vi "Morse Code Decoder.vi"(8 "error in":errorcluster, 10 "Map":map{string, string}(c390), 11 "Message to Decode":string) -> (0 "error out":errorcluster, 3 "Decoded Array":string[](array[string]))   [LabVIEW 2022 SP3]
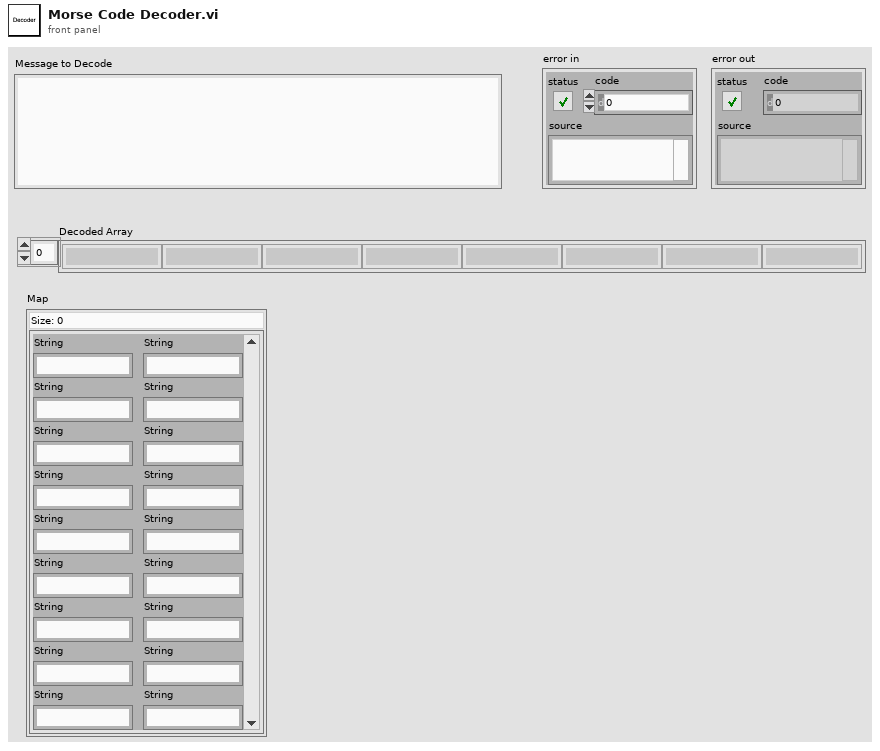
[diagram p1: front panel]
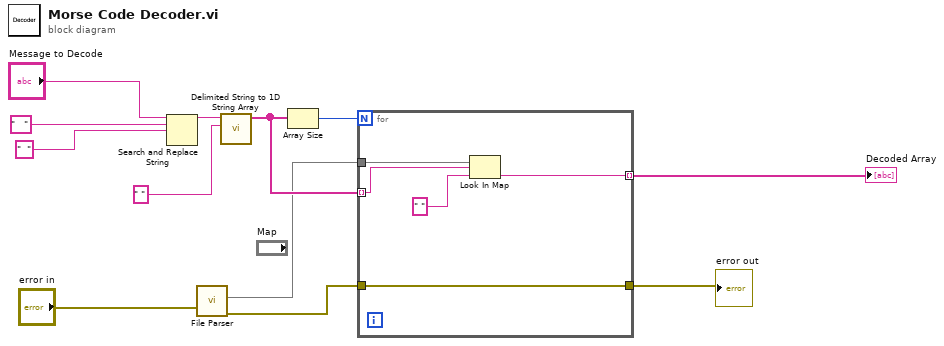
[diagram p0: block diagram]
diagram:
  n1 = Search and Replace String(input string="Message to Decode", search string="   " ("substring (\"\")"), replace string="  " ("replace string (\"\")")) -> (result string=w8:string)  [unwired: 5 in, 3 out]
  n2 = call "File Parser.vi"("error in (no error)"="error in") -> ("error out"=w3:errorcluster, "Morse-Letter Map (output 2)"=w4:map{string, string})  [unwired: 8 in, 1 out]
  n3 = call <vilib>:"Delimited String to 1D String Array.vi"("delimiter"=" ", "delimited string"=w8) -> ("string array"=w6:string[])  [unwired: 9 in]
  n4 = Array Size(array=w6) -> (size(s)=w7:i32)
  n5 = for {
    N: w7 -> [_]
    tunnel: w4 -> [w17]
    tunnel: w6 -> [w16] mode=indexing
    tunnel: [w14] -> w5 mode=indexing
    tunnel: [w13] -> w2
    tunnel: w3 -> [w13]
    n6 = Look In Map(map=w17, key=w16, default value=" ") -> (value=w14:string)  [unwired: 1 out]
  }
  "Decoded Array" <- w5
  "error out" <- w2
